vi "_setAnything.vi"(8 "Error In":errorcluster, 9 "value":variant, 10 "name":string, 11 "DB Ref":T1) -> (0 "Error Out":errorcluster, 1 "created?":bool, 3 "DB Ref(dup)":T1)   [LabVIEW 2014, in "TagDB(dev).lvlib"]
doc: "[Covers: REQ_TAGDB_TEMPLATE_SETVALUE]"
uses:
  TagDB(dev).lvlib
  tagDB_Def.ctl
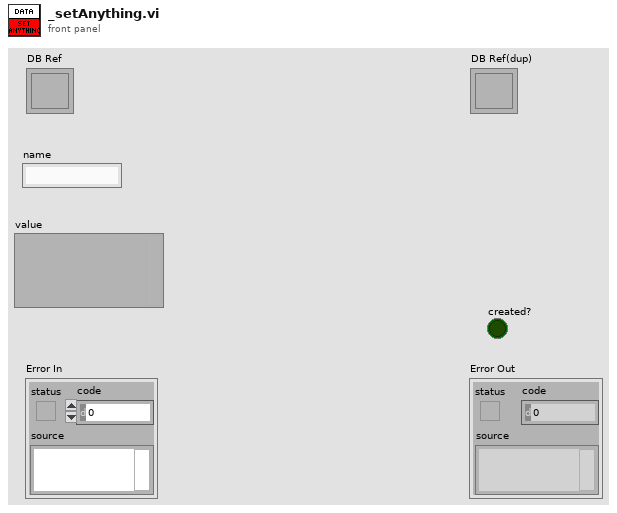
[diagram p1: front panel]
types:
  T1 = typedef "TagDB(dev).lvlib/tagDB_Def.ctl" = refnum<k1>
  T2 = enum8{"Generic", "Datalog File Refnum", "Byte Stream File Refnum", "Device Refnum", "Occurence Refnum", "TCP Connection Refnum", "VISA Refnum (Obsolete)", "Automation Renum", "VI Server Refnum", "Menu Refnum", "IVI Refnum (Obsolete)", "IMAQ Session", "0x0C", "Datasocket Refnum", "VISA Resource", "IVI Logical Name", "UDP Connection Refnum", "Notifier Refnum", "Queue Refnum", "IrDA Refnum", "Hardware Plugin Refnum", "Hardware Plugin Tag Refnum", "DAQmx Refnum", "Event Registration Refnum", ".NET Refnum", "User Event Refnum", "0x1A", "Event Callback", "0x1C", "0x1D", "Only Used Internal to LabVIEW", "Bluetooth", "Data Value References", "RT FIFO", "TDM Streaming"}
  T3 = enum8{"<Null>", "I8", "I16", "I32", "I64", "U8", "U16", "U32", "U64", "SGL", "DBL", "EXT", "CSG", "CDB", "CXT", "0x0F", "0x10", "0x11", "0x12", "0x13", "0x14", "Enum U8", "Enum U16", "Enum U32", "Enum U64", "SGL PQ", "DBL PQ", "EXT PQ", "CSG PQ", "CDB PQ", "CXT PQ", "0x1F", "0x20", "Boolean", "0x22", "0x23", "0x24", "0x25", "0x26", "0x27", "0x28", "0x29", "0x2A", "0x2B", "0x2C", "0x2D", "0x2E", "0x2F", "String", "0x31", "Path", "Pict", "0x34", "0x35", "0x36", "DAQ", "0x38", "0x39", "0x3A", "0x3B", "0x3C", "0x3D", "0x3E", "0x3F", "Array", "0x41", "0x42", "0x43", "0x44", "0x45", "0x46", "0x47", "0x48", "0x49", "0x4A", "0x4B", "0x4C", "0x4D", "0x4E", "0x4F", "Cluster", "0x51", "0x52", "Variant", "Waveform", "0x55", "0x56", "0x57", "0x58", "0x59", "0x5A", "0x5B", "0x5C", "0x5D", "0x5E", "0x5F", "0x60", "0x61", "0x62", "0x63", "0x64", "0x65", "0x66", "0x67", "0x68", "0x69", "0x6A", "0x6B", "0x6C", "0x6D", "0x6E", "0x6F", "Refnum"}
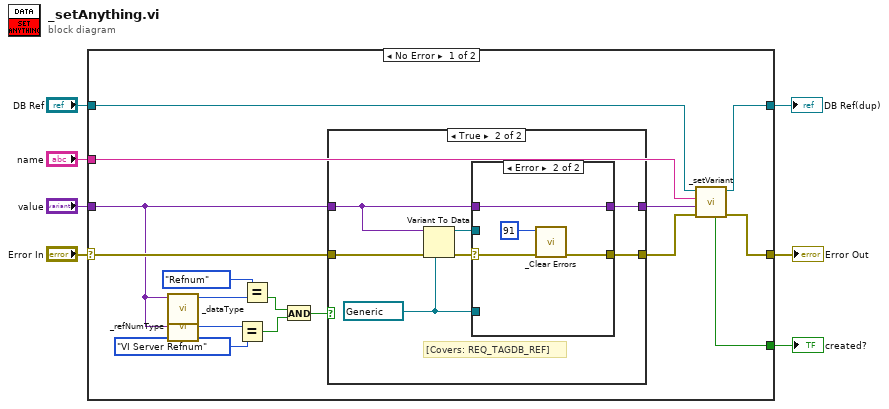
[diagram p0: block diagram]
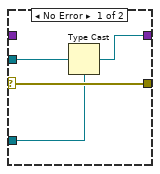
[diagram p3: hidden frame]
diagram:
  n1 = case shown="No Error" "Error In" {
    selector: "Error In" -> [w16 w42]
    tunnel: [w23 w42] -> w7
    tunnel: "DB Ref" -> [w22 w41]
    tunnel: [w21 w41] -> w5
    tunnel: "name" -> [w20 _]
    tunnel: [w19 _] -> w3
    tunnel: "value" -> [w11 _]
    frame No Error {
      n2 = call "_dataType.vi"("Type"=w11) -> ("type"=w15:T3)  [unwired: 10 in]
      n3 = call "_refNumType.vi"("Data"=w11) -> ("Refnum Subtype Enum"=w10:T2)  [unwired: 4 in]
      n4 = Equal?(x=w10, y=T2."VI Server Refnum") -> (x = y?=w9:bool)
      n5 = Equal?(x=T3."Refnum", y=w15) -> (x = y?=w13:bool)
      n6 = And(x=w13, y=w9) -> (x .and. y?=w12:bool)
      n7 = case shown="True" w12 {
        tunnel: w11 -> [w25 w26]
        tunnel: [w25 w30] -> w18
        tunnel: [w24 w27] -> w17
        tunnel: w16 -> [w24 w32]
        frame False {
        }
        frame True {
          w29 = refnum<vi> refnum ("value")
          # "[Covers: REQ_TAGDB_REF]"
          n8 = Variant To Data(error in=w32, type=w29, Variant=w26) -> (data=w31:refnum<vi>, error out=w28:errorcluster)
          n9 = case shown="Error" w28 {
            selector: w28 -> [w36 w39]
            tunnel: w31 -> [w35 _]
            tunnel: [w33 w40] -> w30
            tunnel: w29 -> [w34 _]
            tunnel: [w36 w38] -> w27
            tunnel: w26 -> [_ w40]
            frame No Error {
              n10 = Type Cast(type=w34, x=w35) -> (*(type *) &x=w33:refnum<vi>)
            }
            frame Error {
              n11 = call "_Clear Errors.vi"("error in (no error)"=w39, "specific error code to clear (0: all)"=91) -> ("error out"=w38:errorcluster)  [unwired: 4 in, 1 out]
            }
          }
        }
      }
      n12 = call "_setVariant.vi"("error in (no error)"=w17, "value"=w18, "name"=w20, "DB Ref"=w22) -> ("error in (no error) (dup)"=w23:errorcluster, "DB Ref (dup)"=w21:T1, "created?"=w19:bool)  [unwired: 5 in]
    }
    frame Error {
    }
  }
  "Error Out" <- w7
  "DB Ref(dup)" <- w5
  "created?" <- w3
